vi "WS1021 CS 3 Voltages Output.vi"(8 "Error In":errorcluster, 11 "Data In":string[][](array[string])) -> (0 "Error Out":errorcluster, 1 "3V Vcs Data":string[][](array[string]), 2 "0V Vcs Data":string[][](array[string]), 3 "-3V Vcs Data":string[][](array[string]), 5 "Data Out":string[][](array[string]))   [LabVIEW 2017]
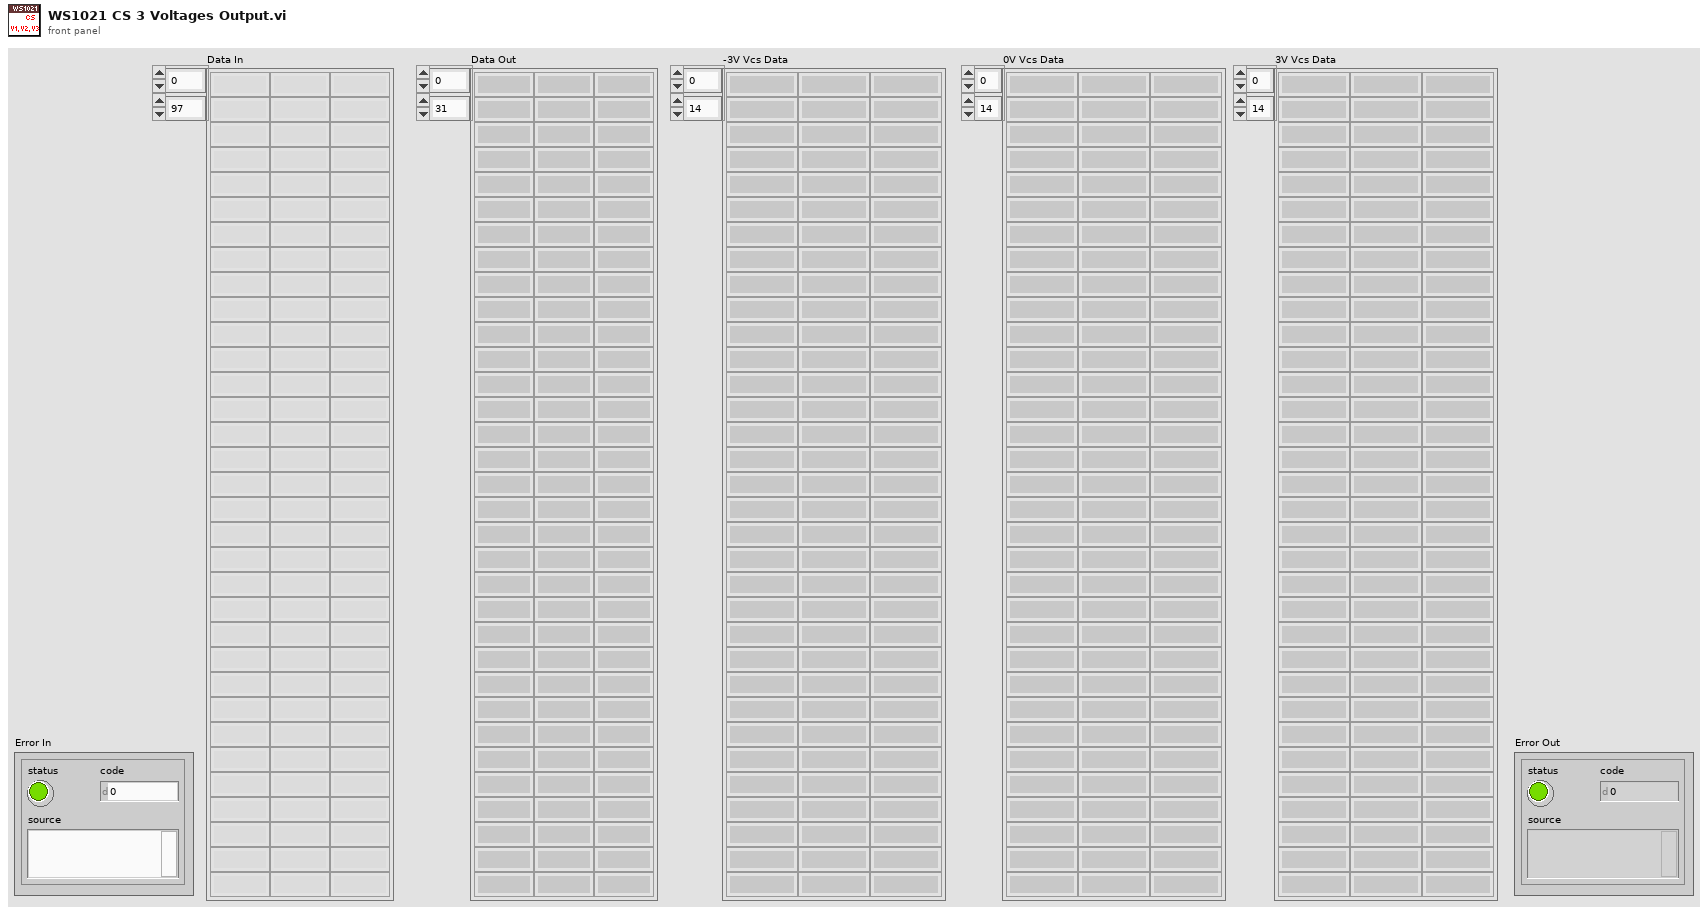
[diagram p1: front panel]
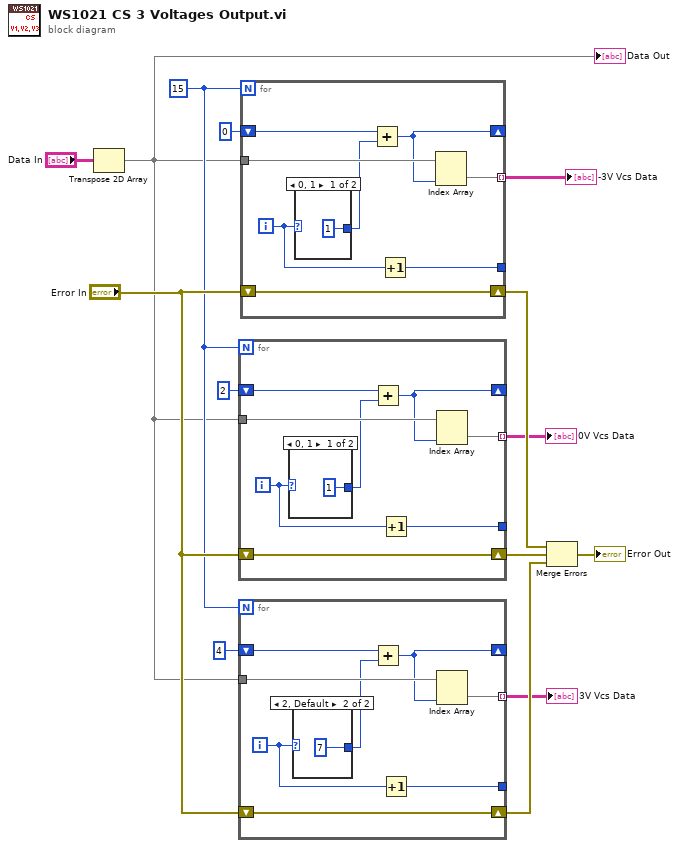
[diagram p0: block diagram]
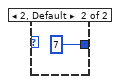
[diagram p2: hidden frame]
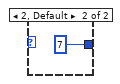
[diagram p3: hidden frame]
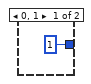
[diagram p4: hidden frame]
diagram:
  w4 = 15
  n1 = Transpose 2D Array(2D array="Data In") -> (transposed array=w1:string[][])
  "Data Out" <- w1
  n2 = for {
    N: w4 -> [_]
    tunnel: w1 -> [w22]
    shift-right: [w19] -> _
    shift-left: 2 -> [w21]
    tunnel: [w18] -> w6 mode=indexing
    tunnel: [w16] -> _
    shift-right: [w15] -> w9
    shift-left: "Error In" -> [w15]
    i -> [w17]
    n3 = case shown="0, 1" w17 {
      tunnel: [1 7] -> w20
      frame 0, 1 {
      }
      frame 2, Default {
      }
    }
    n4 = Add(x=w21, y=w20) -> (x+y=w19:i32)
    n5 = Increment(x=w17) -> (x+1=w16:i32)
    n6 = Index Array(array=w22, index (col)=w19) -> (element=w18:string[])  [unwired: 1 in]
  }
  "0V Vcs Data" <- w6
  n7 = for {
    N: w4 -> [_]
    tunnel: w1 -> [w32]
    shift-right: [w29] -> _
    shift-left: 4 -> [w31]
    tunnel: [w28] -> w5 mode=indexing
    tunnel: [w26] -> _
    shift-right: [w25] -> w8
    shift-left: "Error In" -> [w25]
    i -> [w27]
    n8 = case shown="2, Default" w27 {
      tunnel: [1 7] -> w30
      frame 0, 1 {
      }
      frame 2, Default {
      }
    }
    n9 = Add(x=w31, y=w30) -> (x+y=w29:i32)
    n10 = Increment(x=w27) -> (x+1=w26:i32)
    n11 = Index Array(array=w32, index (col)=w29) -> (element=w28:string[])  [unwired: 1 in]
  }
  "3V Vcs Data" <- w5
  n12 = for {
    N: w4 -> [_]
    tunnel: w1 -> [w42]
    shift-right: [w39] -> _
    shift-left: 0 -> [w41]
    tunnel: [w38] -> w3 mode=indexing
    tunnel: [w36] -> _
    shift-right: [w35] -> w10
    shift-left: "Error In" -> [w35]
    i -> [w37]
    n13 = case shown="0, 1" w37 {
      tunnel: [1 7] -> w40
      frame 0, 1 {
      }
      frame 2, Default {
      }
    }
    n14 = Add(x=w41, y=w40) -> (x+y=w39:i32)
    n15 = Increment(x=w37) -> (x+1=w36:i32)
    n16 = Index Array(array=w42, index (col)=w39) -> (element=w38:string[])  [unwired: 1 in]
  }
  "-3V Vcs Data" <- w3
  n17 = Merge Errors(w10, w9, w8) -> (→"Error Out":errorcluster)
